vi "api_CreateDVR.vi"(8 "error in (no error)":errorcluster, 11 "ConfigClass.lvlib:ConfigClass.lvclass":refnum<class "ConfigClass.lvclass">) -> (0 "error out":errorcluster, 3 "data value reference":refnum<data-value>)   [LabVIEW 2019, in "ConfigClass.lvlib" / "ConfigClass.lvclass"]
uses:
  ConfigClass.lvclass
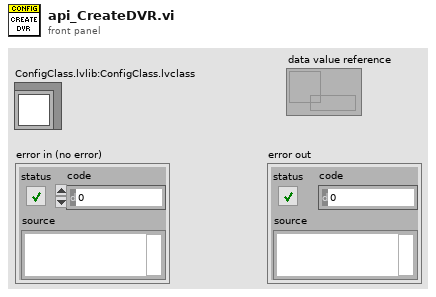
[diagram p1: front panel]
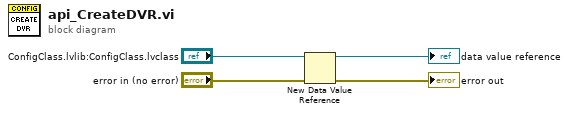
[diagram p0: block diagram]
diagram:
  n1 = New Data Value Reference(data value="ConfigClass.lvlib:ConfigClass.lvclass", error in="error in (no error)") -> (data value reference=→"data value reference":refnum<data-value>, error out=→"error out":errorcluster)
